vi "GPIB-VISA-RW.vi"() -> ()   [LabVIEW 2009]
doc: "This example requires NI-488.2 and NI-VISA to be installed on the system. The example shows how to communicate with a GPIB instrument using VISA reads, writes, and formatting functions on the returned data. This example will work using an NI Instrument Simulator or other instrument that has similar behavior."
uses:
  <vilib>/Instr/_visa.llb/VISA Open Access Mode.ctl
panel:
  in  "VISA resource name":refnum<visa-resource-name>
  out "Read Buffer":string
  in  "Write Buffer":string="SENS:DATA?"
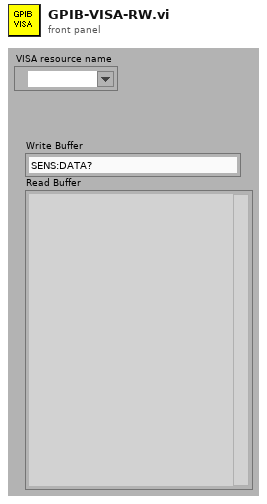
[diagram p1: front panel]
types:
  T1 = typedef "VISA Open Access Mode.ctl" = u32
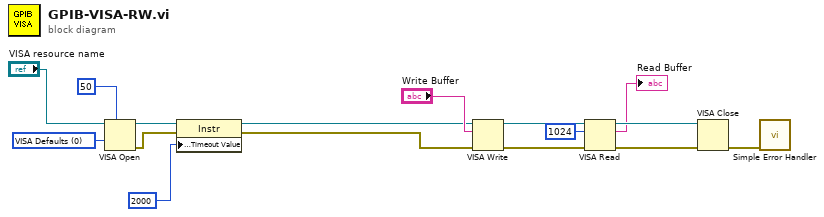
[diagram p0: block diagram]
diagram:
  w8 = T1 0 items=["VISA Defaults"=0, "Exclusive Lock"=1, "Load Configured Settings"=4] ("Access Mode")
  n1 = VISA Open(timeout (0)=u32 50 ("VISA Open timeout (0)"), access mode=w8, VISA resource name="VISA resource name") -> (VISA resource name=w10:refnum<visa-resource-name>, error out=w9:errorcluster)  [unwired: 2 in]
  n2 = property class="Instr"(reference=w10, error in=w9, "General Settings:Timeout Value"=u32 2000) -> (reference out=w2:refnum<visa-resource-name>, error out=w3:errorcluster)
  n3 = VISA Write(VISA resource name=w2, write buffer="Write Buffer", error in (no error)=w3) -> (VISA resource name out=w16:refnum<visa-resource-name>, error out=w14:errorcluster)  [unwired: 1 out]
  n4 = VISA Read(VISA resource name=w16, byte count=u32 1024, error in (no error)=w14) -> (VISA resource name out=w15:refnum<visa-resource-name>, read buffer=→"Read Buffer":string, error out=w13:errorcluster)  [unwired: 1 out]
  n5 = VISA Close(VISA resource name=w15, error in (no error)=w13) -> (error out=w5:errorcluster)
  n6 = call <vilib>:"Simple Error Handler.vi"("error in (no error)"=w5) -> ()  [unwired: 4 in, 5 out]
